vi "Variant to U64 Ary.vi"(10 "Variant":variant) -> (2 "Array":u64[](array[numeric]))   [LabVIEW 2019, in "Variant Parser.lvlib" / "Variant Parser.lvclass"]
uses:
  Library/Variant Parser.lvclass
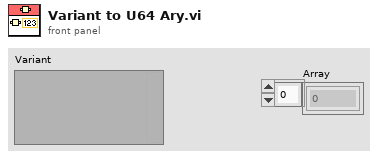
[diagram p1: front panel]
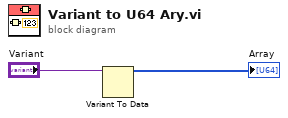
[diagram p0: block diagram]
diagram:
  n1 = Variant To Data(Variant="Variant") -> (data=→"Array":u64[])  [unwired: 2 in, 1 out]
